vi "Run Action.vi"(8 "error in (no error)":errorcluster, 10 "Package":refnum<class "PackageAbstract.lvclass">, 11 "AddAction in":refnum<class "AddAction.lvclass">) -> (0 "error out":errorcluster, 2 "Problems":string[](array[string]), 3 "AddAction out":refnum<class "AddAction.lvclass">)   [LabVIEW 2020, in "GPackTools.lvlib" / "AddAction.lvclass"]
uses:
  AddAction.lvclass
  GPack/PackageAbstract/PackageAbstract.lvclass
  AddAction.lvclass/AddAction.ctl
  InstallAction/InstallAction.lvclass
  <vilib>/regexp/Match Regular Expression.xnode
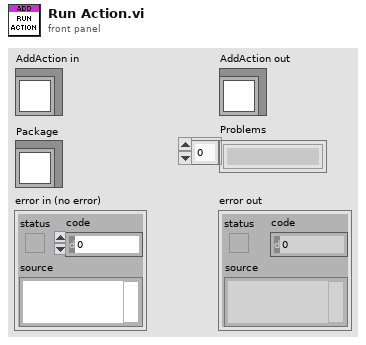
[diagram p1: front panel]
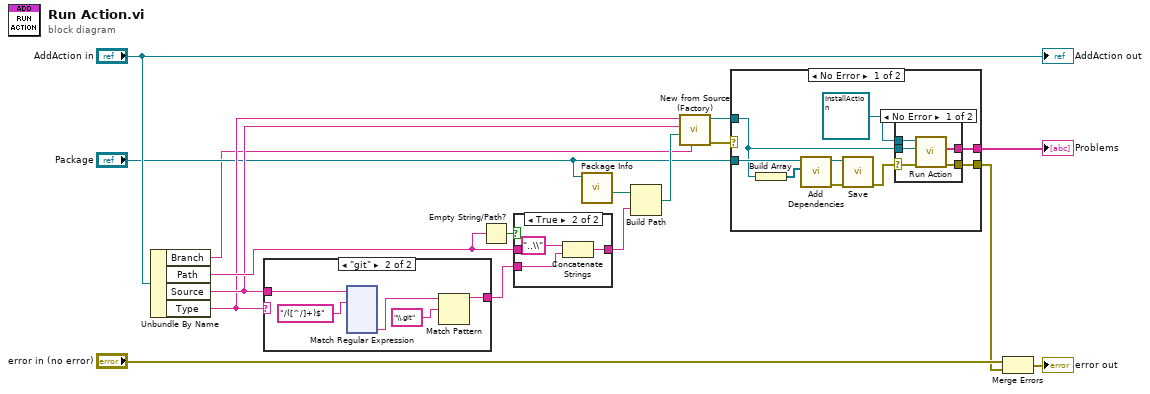
[diagram p0: block diagram]
diagram:
  n1 = Unbundle By Name("AddAction in") -> ("Branch"=w4:string, "Path"=w14:string, "Source"=w10:string, "Type"=w9:string)
  n2 = case shown="\"git\"" w9 {
    tunnel: w10 -> [_ w22]
    tunnel: [_ w18] -> w13
    frame Default {
    }
    frame "git" {
      n3 = xnode "Match Regular Expression"("input string"=w22, "regular expression"="/([^/]+)$") -> ("submatch 1"=w20:string)  [unwired: 4 in, 5 out]
      n4 = Match Pattern(string=w20, regular expression="\\.git") -> (before substring=w18:string)  [unwired: 1 in, 3 out]
    }
  }
  n5 = Empty String/Path?(string/path=w14) -> (empty?=w15:bool)
  n6 = case shown="True" w15 {
    tunnel: w13 -> [_ w141]
    tunnel: w14 -> [w139 _]
    tunnel: [w139 w140] -> w11
    frame False {
    }
    frame True {
      n7 = Concatenate Strings("..\\" ("string"), w141) -> (w140:string)
    }
  }
  n8 = call-dynamic "Package Info.vi"("Package in"="Package") -> ("Folder"=w12:path)  [unwired: 8 in, 2 out]
  n9 = Build Path(base path=w12, name or relative path=w11) -> (appended path=w8:path)
  n10 = call "New from Source (Factory).vi"("Branch (Default)"=w4, "Folder"=w8, "Source"=w10, "Type"=w9) -> ("error out"=w7:errorcluster, "PackageAbstract out"=w5:refnum<class "PackageAbstract.lvclass">)  [unwired: 6 in]
  n11 = case shown="No Error" w7 {
    selector: w7 -> [_ w158]
    tunnel: "Package" -> [w151 _]
    tunnel: w5 -> [w147 _]
    tunnel: [w145 w158] -> w2
    tunnel: [w143 _] -> w1
    frame No Error {
      n12 = Build Array(w147) -> (w150:refnum<class "PackageAbstract.lvclass">[])
      n13 = call "Add Dependencies.vi"("Dependencies"=w150, "PackageAbstract in"=w151) -> ("error out"=w148:errorcluster, "PackageAbstract out"=w149:refnum<class "PackageAbstract.lvclass">)  [unwired: 8 in]
      n14 = call "Save.vi"("error in (no error)"=w148, "PackageAbstract in"=w149) -> ("error out"=w146:errorcluster)  [unwired: 8 in, 1 out]
      n15 = case shown="No Error" w146 {
        selector: w146 -> [w156 w157]
        tunnel: w147 -> [w154 _]
        tunnel: [w155 w157] -> w145
        tunnel: refnum<class "InstallAction.lvclass"> refnum ("GPackTools.lvlib:InstallAction.lvclass") -> [w153 _]
        tunnel: [w152 _] -> w143
        frame No Error {
          n16 = call-dynamic "Run Action.vi"("error in (no error)"=w156, "Package"=w154, "InstallAction in"=w153) -> ("error out"=w155:errorcluster, "Problems"=w152:string[])  [unwired: 6 in, 1 out]
        }
        frame Error {
        }
      }
    }
    frame Error {
    }
  }
  "Problems" <- w1
  n17 = Merge Errors("error in (no error)", w2) -> (→"error out":errorcluster)
  "AddAction out" <- "AddAction in"
